vi "PockelsControl.vi"(8 "Error In":errorcluster, 10 "Laser Power (%)":dbl max=100.0 step=1.0) -> (0 "Error Out":errorcluster)   [LabVIEW 2020]
uses:
  Peripherals Control/Shutter/Typedefs/Shutter state.ctl
  Typedefs/HW config states enum.ctl
  Typedefs/Imaging Protocols enum.ctl
  <vilib>/DAQmx/write.llb/DAQmx Write (Analog DBL 1Chan 1Samp).vi
  Global Variables/General Globals.vi
  Peripherals Control/Pockels/Globals/gl_Pockels control globals.vi
  <vilib>/DAQmx/create/channels.llb/DAQmx Create Channel (AO-Voltage-Basic).vi
  <vilib>/DAQmx/miscellaneous.llb/DAQmx Fill In Error Info.vi
  Global Variables/gl_UI Ctrl Refs.vi
panel:
  out "DAQmx Physical Channel":tag="PXI1Slot4/ao0"
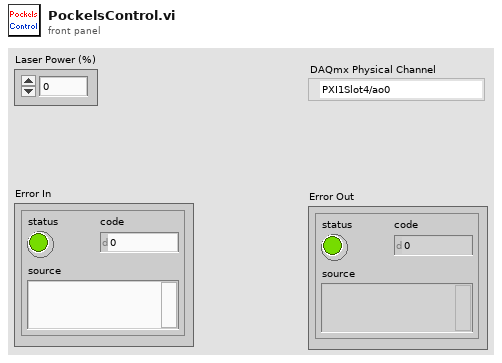
[diagram p1: front panel]
types:
  T1 = typedef "HW config states enum.ctl" = enum16{"Load from file", "Save to file", "Save backup", "Write all", "Read all", "Write XY stage settings", "Write DAQ FPGA settings", "Write Control FPGA settings", "Write Phys Channels", "Write System Config", "Write HW Config", "Save System Config", "Save HW Config", "Clear", "Compare from file"}
  T2 = typedef "Shutter state.ctl" = enum16{"Closed/Disabled", "Open/Enabled"}
  T3 = typedef "Hardware Configuration settings.ctl" = cluster{"Dev. PC":bool, "Swap XY on stage":bool, "No of AOD":u8, "MC Supported":bool, "Axial MC":bool, "Computer MAC address":string, "Externalise Triggers":bool, "Trigger HW config":T4, "DAQmx Chan":T5, "XY stage available":bool, "XY Stage":T6, "Z stage available":bool, "Z Stage config cluster":T7, "Encoder available":bool, "Encoder":T8, "VidRec available":bool, "Cam VidRec":T9, "Laser Power Control HW config":T10, "Laser 1 available":bool, "Laser 1 config cluster":T11, "Prechirper 1 available":bool, "Prechirper 1 config cluster":T12, "Control system.FPGA available?":bool, "Control Sys. HW config":T13, "DAQ FPGA HW Config":T14, "PMT Voltage Range":T18}
  T4 = typedef "Triggers HW config.ctl" = cluster{"Available Device List":i32, "Device Address":string}
  T5 = typedef "DAQmx physical channels cluster.ctl" = cluster{"Pockels AO":tag, "Hard shutter AO":tag, "PMT AOs":tag, "Galvo AOs":tag, "Power meter AI":tag}
  T6 = typedef "XY Stage config cluster.ctl" = cluster{"COM port":refnum<visa-resource-name>, "Baudrate":i32, "Type":string}
  T7 = typedef "Z Stage config cluster.ctl" = cluster{"COM port":refnum<visa-resource-name>, "Baudrate":i32, "Type":string}
  T8 = typedef "Encoder config cluster.ctl" = cluster{"IP address":string, "Port":u16, "Wheel radius (cm)":dbl, "Encoder Trigger":tag}
  T9 = typedef "Cam VidRec HW config setup cluster.ctl" = cluster{"DO flag-Video record":tag, "DO flag-Trial start":tag}
  T10 = typedef "Laser Power Control HW config.ctl" = cluster{"Laser Power Control":string, "Laser Power Modulation Control":enum16{"NI", "FPGA"}}
  T11 = typedef "Laser 1 config cluster.ctl" = cluster{"COM port":refnum<visa-resource-name>, "Baud Rate":i32, "Type":string}
  T12 = typedef "PreChirper 1 config cluster.ctl" = cluster{"Type":string, "Baud Rate":i32, "COM port":refnum<visa-resource-name>}
  T13 = typedef "Control Sys HW config cluster.ctl" = cluster{"Control system.FPGA Type":enum16{"Virtex 5", "Virtex 7"}, "Control system.Network adapter name":string, "Control system.MAC address":string, "Control system.Ethernet Port":u32, "Control system.Ethernet Port Opened":bool}
  T14 = typedef "DAQ FPGA HW config cluster.ctl" = cluster{"FGPA Ref":T15, "Target":T16, "input card type":T17}
  T15 = typedef "FPGA Ref.ctl" = refnum<k20>
  T16 = typedef "nirio_resource_hc.ctl" = tag
  T17 = typedef "FPGA input type AC-DC.ctl" = enum16{"AC Card", "DC Card"}
  T18 = typedef "PMT Voltage Range.ctl" = cluster{"PMT Voltage Lower Limit":dbl, "PMT Voltage Upper Limit":dbl}
  T19 = enum8{"Clear the register", "Always ON", "Modulate"}
  T20 = typedef "Imaging Protocols enum.ctl" = enum16{"AOL Z-Stack", "Motor Z Stack", "Functional Acquisition", "Single Plane Acquisition", "Volume Acquisition", "Live Imaging", "Live Plane Imaging", "Live Volume Imaging"}
  T21 = typedef "UI ctrl refs cluster.ctl" = cluster{"Top level VI path":path, "Top level VI ref":refnum<vi>, "User menu ref":refnum<k9>, "Sub Panel control":refnum<vi>, "Imaging Param Tab":refnum<vi>, "Occurrence-Start drivers":refnum<k4>, "Occurrence-Speed logging initialised":refnum<k4>, "Occurrence-XYZ stage initialised":refnum<k4>, "Exit button":refnum<vi>, "Status ind":refnum<vi>, "Set as origin":refnum<vi>, "Speed Logging":refnum<vi>, "Time Lapse":refnum<vi>, "Live Imaging":refnum<vi>, "AOL Z Stack":refnum<vi>, "Motor Z Stack":refnum<vi>, "Funct Acq button":refnum<vi>, "Hard Shutter":refnum<vi>, "Virtual Shutter":refnum<vi>, "Laser Power":refnum<vi>, "AOL Mode":refnum<vi>, "Frame Size":refnum<vi>, "Field of View":refnum<vi>, "Dwell Time":refnum<vi>, "Zoom":refnum<vi>, "AOL Z":refnum<vi>, "Objective":refnum<vi>, "Axis":refnum<vi>, "Paths & Names":refnum<vi>, "Experiment folder path (ind.)":refnum<vi>, "Last State (Ind.)":refnum<vi>, "Averages":refnum<vi>, "Angle (degrees)":refnum<vi>, "X centre":refnum<vi>, "Y centre":refnum<vi>, "Plane Mode":refnum<vi>, "# Planes":refnum<vi>, "Z Start":refnum<vi>, "Z Stop":refnum<vi>, "Z Step":refnum<vi>, "PMT 1":refnum<vi>, "PMT 2":refnum<vi>, "Stage XYZ Position":refnum<vi>, "Pockels@Z Start":refnum<vi>, "Pockels@Z Stop":refnum<vi>, "Obtain Z Start":refnum<vi>, "Obtain Z Stop":refnum<vi>, "Live stim.trig.period":refnum<vi>, "Live stim.trig.enable":refnum<vi>, "Movement Correction":refnum<vi>, "Load Reference Image":refnum<vi>, "XY Stage Move":refnum<vi>, "MovCor Cluster":refnum<vi>, "RefDAQParam":refnum<vi>, "Funct. Acq. Pockels Modulation":refnum<vi>, "Ref Laser Power":refnum<vi>, "Enable Video Recording":refnum<vi>, "Video Record-Live Imaging":refnum<vi>, "Video Record-Funct acq":refnum<vi>, "Reference Source":refnum<vi>, "AOL Z-stack Chirps Ready (ind)":refnum<vi>, "Target time between mov.cor. ref triggers (ms)":refnum<vi>, "Funct. Acq. Ref frame save":refnum<vi>, "Tracking button":refnum<vi>, "Show ref plots window":refnum<vi>, "Center freq ind (nm)":refnum<vi>, "Pickup mode (ind)":refnum<vi>, "Logging queue (ind)":refnum<vi>, "Back aperture power (ind.)":refnum<vi>, "Power after objective (ind.)":refnum<vi>, "Switch user":refnum<vi>, "Ls1 Conn. Status":refnum<vi>, "Ls1Tuning Status":refnum<vi>, "Ls1 Faults":refnum<vi>, "Ls1 Connection":refnum<vi>, "Ls1 Mode":refnum<vi>, "Ls1 POWER [mW]":refnum<vi>, "Ls1Shutter":refnum<vi>, "Ls1 Wavelength":refnum<vi>, "Ls1 Note":refnum<vi>, "Ls1 Confirm Wav":refnum<vi>, "Ls1 PreChrp Prism1":refnum<vi>, "Ls1 PreChrp Prism2":refnum<vi>, "Ls1 wav top Ind":refnum<vi>, "Ls1 power top Ind":refnum<vi>, "Ls1 Pump peak Hold":refnum<vi>, "Ls1 Status Ind":refnum<vi>, "Ls1 wav cancel":refnum<vi>, "Experiment Type":refnum<vi>, "Biology Information":refnum<vi>, "Camera recording status":refnum<vi>}
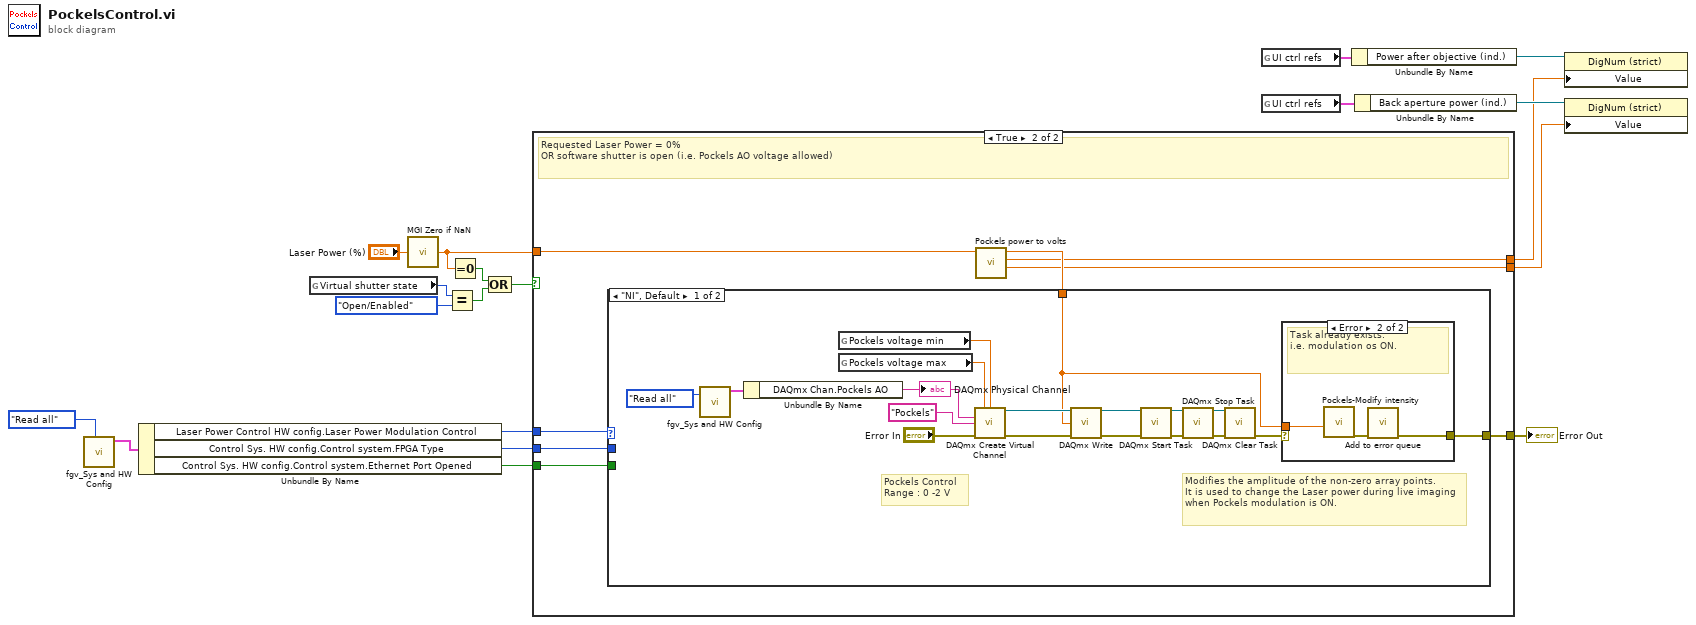
[diagram p0: block diagram]
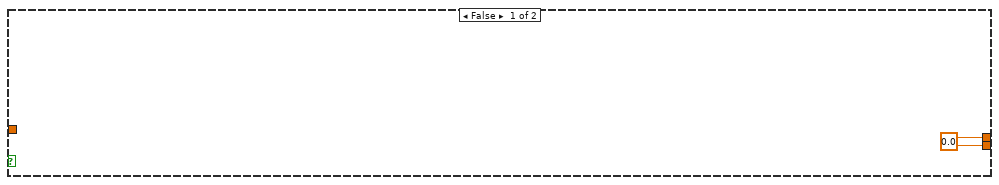
[diagram p2: hidden frame]
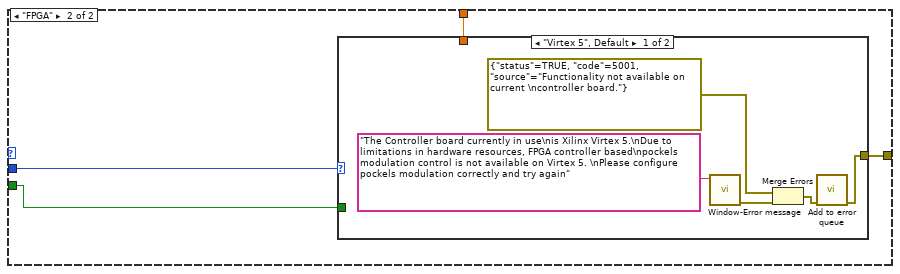
[diagram p4: hidden frame]
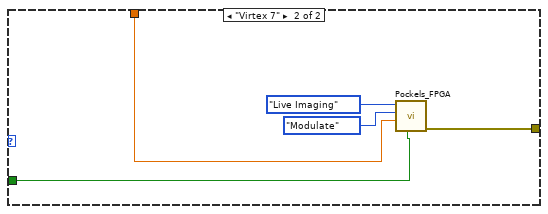
[diagram p5: hidden frame]
diagram:
  n1 = call "fgv_Sys and HW Config.vi"("Function"=HW_config_states_enum."Read all") -> ("Hardware Configuration OUT"=w4:T3)  [unwired: 8 in, 2 out]
  n2 = Unbundle By Name(w4) -> ("Laser Power Control HW config.Laser Power Modulation Control"=w3:enum16{"NI", "FPGA"}, "Control Sys. HW config.Control system.FPGA Type"=w2:enum16{"Virtex 5", "Virtex 7"}, "Control Sys. HW config.Control system.Ethernet Port Opened"=w1:bool)
  n3 = global read "General Globals.vi" "Virtual shutter state"() -> (w15:T2)
  n4 = call <userlib>:"MGI Zero if NaN.vi"("Number In"="Laser Power (%)") -> ("Number Out"=w6:dbl)
  n5 = Equal?(x=w15, y=Shutter_state."Open/Enabled") -> (x = y?=w16:bool)
  n6 = Equal To 0?(x=w6) -> (x = 0?=w17:bool)
  n7 = Compound Arithmetic op=OR(w17, w16) -> (w14:bool)
  n8 = case shown="True" w14 {
    tunnel: [_ w28] -> w19
    tunnel: w6 -> [_ w27]
    tunnel: [w20 w25] -> w11
    tunnel: [w20 w24] -> w8
    tunnel: w3 -> [_ w23]
    tunnel: w2 -> [_ w22]
    tunnel: w1 -> [_ w21]
    frame False {
      w20 = 0.0 ("Normalised power (mW)")
    }
    frame True {
      # "Requested Laser Power = 0%\nOR software shutter is open (i.e. Pockels AO voltage allowed)"
      n9 = call "Pockels power to volts.vi"("Pockels power (%)"=w27) -> ("Back-aperture power (mW)"=w25:dbl, "Power after the objective (mW)"=w24:dbl, "Pockels control voltage (V)"=w26:dbl)  [unwired: 8 in]
      n10 = case shown="\"NI\", Default" w23 {
        tunnel: [w36 w53] -> w28
        tunnel: w26 -> [w32 w52]
        tunnel: w22 -> [_ w51]
        tunnel: w21 -> [_ w50]
        frame "NI", Default {
          # "Modifies the amplitude of the non-zero array points.\nIt is used to change the Laser power during live imaging when Pockels modulation is ON."
          # "Pockels Control\nRange : 0 -2 V"
          n11 = call "fgv_Sys and HW Config.vi"("Function"=HW_config_states_enum."Read all") -> ("Hardware Configuration OUT"=w30:T3)  [unwired: 8 in, 2 out]
          n12 = Unbundle By Name(w30) -> ("DAQmx Chan.Pockels AO"=w29:tag)
          "DAQmx Physical Channel" <- w29
          n13 = global read "gl_Pockels control globals.vi" "Pockels voltage min"() -> (w34:dbl)
          n14 = global read "gl_Pockels control globals.vi" "Pockels voltage max"() -> (w33:dbl)
          n15 = call-poly <vilib>:"DAQmx Create Virtual Channel.vi"("maximum value"=w33, "minimum value"=w34, "physical channels"=w29, "name to assign"="Pockels", "error in"="Error In") -> ("task out"=w46:refnum<k21>, "error out"=w45:errorcluster)  [unwired: 9 in]
          n16 = call-poly <vilib>:"DAQmx Write.vi"("task/channels in"=w46, "data"=w32, "error in"=w45) -> ("task out"=w44:refnum<k21>, "error out"=w43:errorcluster)  [unwired: 10 in, 1 out]
          n17 = call <vilib>:"DAQmx Start Task.vi"("task/channels in"=w44, "error in"=w43) -> ("task out"=w37:refnum<k21>, "error out"=w38:errorcluster)  [unwired: 12 in]
          n18 = call <vilib>:"DAQmx Stop Task.vi"("task/channels in"=w37, "error in"=w38) -> ("task out"=w42:refnum<k21>, "error out"=w41:errorcluster)  [unwired: 12 in]
          n19 = call <vilib>:"DAQmx Clear Task.vi"("task in"=w42, "error in"=w41) -> ("error out"=w35:errorcluster)  [unwired: 13 in]
          n20 = case shown="Error" w35 {
            tunnel: [_ w47] -> w36
            tunnel: w32 -> [_ w49]
            frame No Error {
            }
            frame Error {
              # "Task already exists.\ni.e. modulation os ON."
              n21 = call "Pockels-Modify intensity.vi"("Pockels control value (V)"=w49) -> ("error out"=w48:errorcluster)  [unwired: 9 in, 1 out]
              n22 = call "Add to error queue.vi"("error in (no error)"=w48) -> ("error out"=w47:errorcluster)  [unwired: 10 in]
            }
          }
        }
        frame "FPGA" {
          n23 = case shown="\"Virtex 5\", Default" w51 {
            tunnel: [w54 w61] -> w53
            tunnel: w52 -> [_ w60]
            tunnel: w50 -> [_ w59]
            frame "Virtex 5", Default {
              n24 = call "Window-Error message.vi"("Message"="The Controller board currently in use\nis Xilinx Virtex 5.\nDue to limitations in hardware resources, FPGA controller based\npockels modulation control is not available on Virtex 5. \nPlease configure pockels modulation correctly and try again") -> ("Error Out (no error)"=w57:errorcluster)  [unwired: 10 in]
              n25 = Merge Errors(errorcluster {"status"=TRUE, "code"=5001, "source"="Functionality not available on current \ncontroller board."} ("error in (no error)"), w57) -> (w55:errorcluster)
              n26 = call "Add to error queue.vi"("error in (no error)"=w55) -> ("error out"=w54:errorcluster)  [unwired: 10 in]
            }
            frame "Virtex 7" {
              n27 = call "Pockels_FPGA.vi"("Ethernet Port Opened ?"=w59, "Laser(V)"=w60, "Pockels Mode_FPGA"=T19."Modulate", "Imaging Protocol"=Imaging_Protocols_enum."Live Imaging") -> ("error out"=w61:errorcluster)  [unwired: 6 in, 1 out]
            }
          }
        }
      }
    }
  }
  "Error Out" <- w19
  n28 = global read "gl_UI Ctrl Refs.vi" "UI ctrl refs"() -> (w9:T21)
  n29 = global read "gl_UI Ctrl Refs.vi" "UI ctrl refs"() -> (w13:T21)
  n30 = Unbundle By Name(w9) -> ("Power after objective (ind.)"=w10:refnum<vi>)
  n31 = Unbundle By Name(w13) -> ("Back aperture power (ind.)"=w12:refnum<vi>)
  n32 = property class="DigNum (strict)"(reference=w10, "Value"=w8) -> ()  [unwired: 1 in, 2 out]
  n33 = property class="DigNum (strict)"(reference=w12, "Value"=w11) -> ()  [unwired: 1 in, 2 out]
